vi "IMAQ FPGA CXP 8-Bit x 16.vi"(6 "Ready for Output":bool=TRUE, 7 "Reset":bool, 9 "Image Skip Count":u16, 10 "CXP Options":T1, 11 "CXP NI AXI4-S Bus":T3) -> (0 "Output Valid":bool, 2 "Acquisition Status":T2, 3 "Vision Pixel Bus Out":T4={"Pixel Data"=[0, 0, 0, 0, 0, 0, 0, 0, 0, 0, 0, 0, 0, 0, 0, 0], "DV"=[FALSE, FALSE, FALSE, FALSE, FALSE, FALSE, FALSE, FALSE, FALSE, FALSE, FALSE, FALSE, FALSE, FALSE, FALSE, FALSE], "EOL"=FALSE, "EOI"=FALSE, "Data Type"=enum."U8 x 16"}, 4 "Ready For Input":bool)   [LabVIEW 2020]
doc: "Acquires images from a CoaXPress camera. The VI converts the pixels from NI_AXI4-S format to Vision Pixel Bus containing 16 adjacent pixels. The <B>Vision Pixel Bus Out</B> can be connected to Vision FPGA algorithms for processing or transferred to the host. Ensure that this VI is called from a Single Cycle Timed Loop. Use multiple instances of this VI along with <B>Device ID</B> and <B>Stream ID</B> inputs to output a Vision Pixel Bus for multiple cameras."
uses:
  <vilib>/visionFPGA/Controls/IMAQ FPGA Pixel Bus u8x16.ctl
  <vilib>/visionFPGA/Basics/CoaXPress Acquisition/Controls/IMAQ FPGA CXP NI AXI4-S Bus.ctl
  <vilib>/visionFPGA/Basics/CoaXPress Acquisition/Controls/IMAQ FPGA CXP FPGA Options.ctl
  <vilib>/rvi/Emulation/niFpgaSctlEmulationGetInTimedLoop.vi
  <vilib>/Utility/error.llb/Clear Errors.vi
  <vilib>/rvi/DataTransferAndStorage/Container/Common/niFpgaContainerGetUniqueNameForEmu.vi
  <vilib>/rvi/DataTransferAndStorage/Container/Common/niFpgaContainerSetEmuInfo.vi
  <vilib>/rvi/eio/common/nirviEmuReportErrorAndStop.vi
  <vilib>/rvi/DataTransferAndStorage/Container/Common/niFpgaContainerExecOnDevCompGetState.vi
  <vilib>/rvi/Emulation/niFpgaEmulationIsFPGAContextNoSignature.vi
  <vilib>/rvi/errors/niFpgaSetErrorForExecOnDevCompSimple.vi
  <vilib>/rvi/FIFO/Fifo_Resource/nirvififoEmulationSetSize.vi
  <vilib>/rvi/FIFO/Fifo_Resource/nirviFifoEmulationQueueMgr.vi
  <instcachedir>/0/nirviFifoEmulationQueueMgr_E5CAEC123FF24DC58D834DCA3CDAA9B5.lvgen/nirviFifoEmulationQueueMgr_E5CAEC123FF24DC58D834DCA3CDAA9B5_008.vi
  <vilib>/rvi/FIFO/Fifo_Resource/nirvififoEmulationDetermineInputValidOut.vi
  <vilib>/rvi/FIFO/Fifo_Resource/nirvififoEmulationCreateLock.vi
  <vilib>/rvi/Emulation/niFpgaProcessEmulError.vi
  <vilib>/rvi/FIFO/Fifo_Resource/nirvififoEmulationObtainLock.vi
  <vilib>/rvi/FIFO/Fifo_Resource/nirvififoEmulationReleaseLock.vi
  <vilib>/rvi/occurrence/nirviWaitOnOccurrenceBase.vi
  <vilib>/rvi/errors/nirviReportUnexpectedCaseInternalError.vi
  <vilib>/rvi/errors/nirviReportUnexpectedCaseInternalError (U32).vi
  <vilib>/rvi/interface/RandomDataEmulation/niFpgaRandomDataHandleErrors.vi
  <vilib>/rvi/LocalResourceManager/LocalResourceManager.xnode
  <vilib>/rvi/DataTransferAndStorage/Container/XNode/niFpgaContainer.xnode
  <vilib>/rvi/FIFO/Fifo_Resource/niFpgaFifoEmulationRefIn.vi
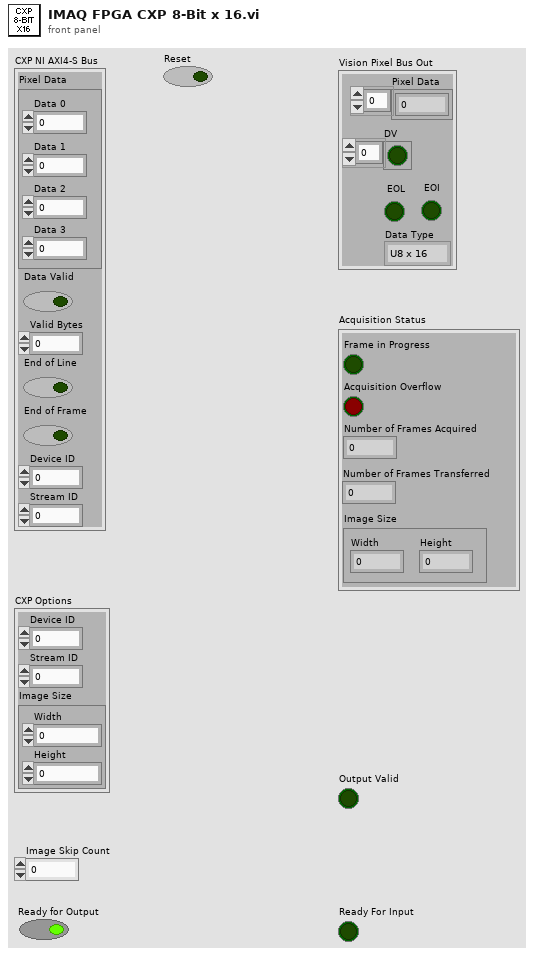
[diagram p1: front panel]
types:
  T1 = typedef "IMAQ FPGA CXP FPGA Options.ctl" = cluster{"Device ID":u8, "Stream ID":u8, "Image Size":cluster{"Width":u16, "Height":u16}}
  T2 = cluster{"Frame in Progress":bool, "Acquisition Overflow":bool, "Number of Frames Acquired":u64, "Number of Frames Transferred":u64, "Image Size":cluster{"Width":u16, "Height":u16}}
  T3 = typedef "IMAQ FPGA CXP NI AXI4-S Bus.ctl" = cluster{"Pixel Data":cluster{"Data 0":u64, "Data 1":u64, "Data 2":u64, "Data 3":u64}, "Data Valid":bool, "Valid Bytes":u8, "End of Line":bool, "End of Frame":bool, "Device ID":u8, "Stream ID":u8}
  T4 = typedef "IMAQ FPGA Pixel Bus u8x16.ctl" = cluster{"Pixel Data":u8[], "DV":bool[], "EOL":bool, "EOI":bool, "Data Type":enum16{"U8 x 16"}}
  T5 = cluster{"Pixel Data":cluster{"Data 0":u64, "Data 1":u64, "Data 2":u64, "Data 3":u64}, "Data Valid":bool, "Valid Bytes":u8, "End of Line":bool, "End of Frame":bool, "Device ID":u8, "Stream ID":u8}
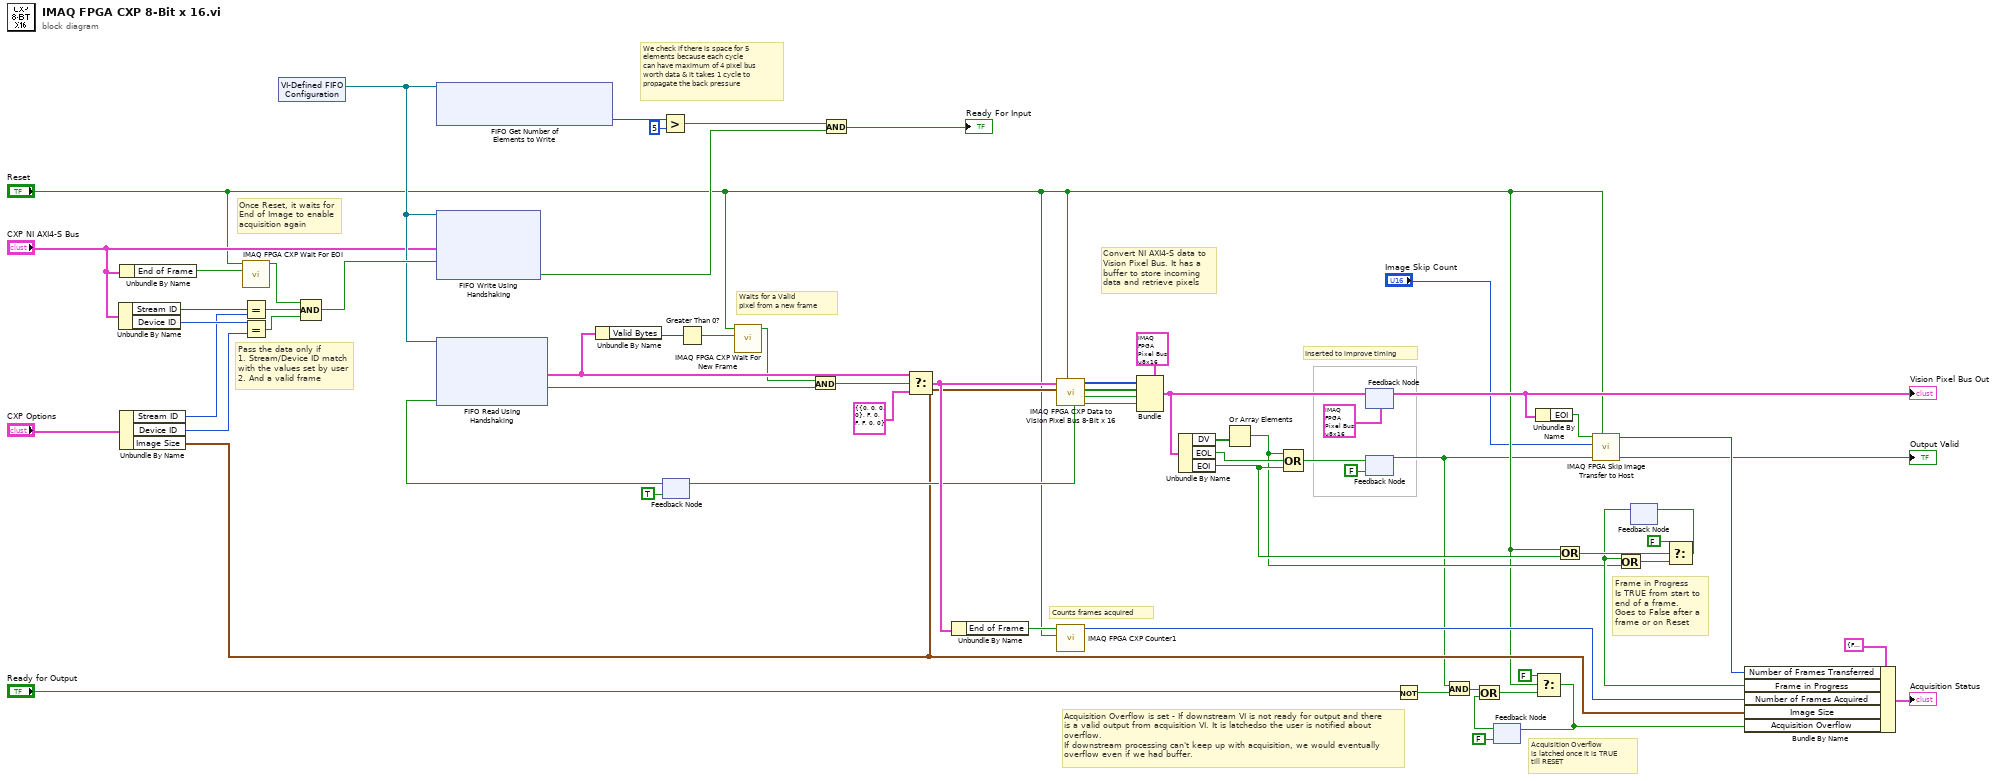
[diagram p0: block diagram]
diagram:
  # "We check if there is space for 5\nelements because each cycle\ncan have maximum of 4 pixel bus\nworth data & it takes 1 cycle to \npropagate the back pressure"
  # "Waits for a Valid\npixel from a new frame"
  # "Pass the data only if\n1. Stream/Device ID match\nwith the values set by user\n2. And a valid frame"
  # "Once Reset, it waits for\nEnd of Image to enable\nacquisition again"
  # "Frame in Progress\nIs TRUE from start to \nend of a frame. \nGoes to False after a\nframe or on Reset"
  # "Acquisition Overflow\nis latched once it is TRUE\ntill RESET"
  # "Convert NI AXI4-S data to\nVision Pixel Bus. It has a \nbuffer to store incoming\ndata and retrieve pixels"
  # "Counts frames acquired"
  # "Inserted to improve timing"
  # "Acquisition Overflow is set - If downstream VI is not ready for output and there \nis a valid output from acquisition VI. It is latchedso the user is notified about\noverflow. \nIf downstream processing can't keep up with acquisition, we would eventually \noverflow even if we had buffer."
  n1 = Unbundle By Name("CXP NI AXI4-S Bus") -> ("Stream ID"=w44:u8, "Device ID"=w43:u8)
  n2 = Unbundle By Name("CXP Options") -> ("Stream ID"=w12:u8, "Device ID"=w11:u8, "Image Size"=w10:cluster{"Width":u16, "Height":u16})
  n3 = Unbundle By Name("CXP NI AXI4-S Bus") -> ("End of Frame"=w23:bool)
  n4 = call <vilib>:"IMAQ FPGA CXP Wait For EOI.vi"("EOI"=w23, "Reset"="Reset") -> ("Enable"=w24:bool)  [unwired: 9 in]
  n5 = Equal?(x=w44, y=w12) -> (x = y?=w53:bool)
  n6 = Equal?(x=w43, y=w11) -> (x = y?=w52:bool)
  n7 = xnode "VI-Defined FIFO Configuration"() -> ("FIFO Out"=w36:refnum<k21>)
  n8 = Compound Arithmetic op=AND(w24, w53, w52) -> (w39:bool)
  n9 = xnode "FIFO Get Number of Elements to Write"("FIFO In"=w36) -> ("Number of Elements to Write"=w37:u32)  [unwired: 1 out]
  n10 = xnode "FIFO Write Using Handshaking"("Element"="CXP NI AXI4-S Bus", "Input Valid"=w39, "FIFO In"=w36) -> ("Ready for Input"=w21:bool)  [unwired: 1 out]
  n11 = Greater?(x=w37, y=u32 5) -> (0:w22:bool)
  n12 = feedback #1(TRUE ("Ready for Input")) -> (w34:bool)
  n13 = xnode "FIFO Read Using Handshaking"("Ready for Output"=w34, "FIFO In"=w36) -> ("Element"=w19:T5, "Output Valid"=w15:bool)  [unwired: 1 out]
  n14 = Unbundle By Name(w19) -> ("Valid Bytes"=w18:u8)
  n15 = Greater Than 0?(x=w18) -> (x > 0?=w17:bool)
  n16 = call <vilib>:"IMAQ FPGA CXP Wait For New Frame.vi"("DV"=w17, "Reset"="Reset") -> ("Enable"=w16:bool)  [unwired: 9 in]
  n17 = And(x=w16, y=w15) -> (x .and. y?=w14:bool)
  n18 = And(x=w22, y=w21) -> (x .and. y?=→"Ready For Input":bool)
  n19 = Select(t=w19, s=w14, f=T3 {"Pixel Data"={"Data 0"=0, "Data 1"=0, "Data 2"=0, "Data 3"=0}, "Data Valid"=FALSE, "Valid Bytes"=0, "End of Line"=FALSE, "End of Frame"=FALSE, "Device ID"=0, "Stream ID"=0} ("CXP NI AXI4-S Bus")) -> (s? t:f=w47:T3)
  n20 = Unbundle By Name(w47) -> ("End of Frame"=w49:bool)
  n21 = call <vilib>:"IMAQ FPGA CXP Data to Vision Pixel Bus 8-Bit x 16.vi"("Reset"="Reset", "Image Size"=w10, "CXP Data"=w47) -> ("EOI"=w61:bool, "EOL"=w62:bool, "DV"=w63:bool[], "Pixel Data"=w64:u8[], "Ready for Input"=w35:bool)  [unwired: 4 in]
  n22 = feedback-in #1(w35) -> ()
  n23 = call <vilib>:"IMAQ FPGA CXP Counter1.vi"("Reset"="Reset", "Increment"=w49) -> ("Count 1"=w48:u64)  [unwired: 9 in]
  n24 = Bundle(cluster=T4 {"Pixel Data"=[0, 0, 0, 0, 0, 0, 0, 0, 0, 0, 0, 0, 0, 0, 0, 0], "DV"=[FALSE, FALSE, FALSE, FALSE, FALSE, FALSE, FALSE, FALSE, FALSE, FALSE, FALSE, FALSE, FALSE, FALSE, FALSE, FALSE], "EOL"=FALSE, "EOI"=FALSE, "Data Type"=enum."U8 x 16"} ("Vision Pixel Bus Out"), "Pixel Data"=w64, "DV"=w63, "EOL"=w62, "EOI"=w61) -> (w60:T4)  [unwired: 1 in]
  n25 = Unbundle By Name(w60) -> ("DV"=w65:bool[], "EOL"=w66:bool, "EOI"=w27:bool)
  n26 = Or Array Elements(Boolean array=w65) -> (logical OR=w26:bool)
  n27 = Compound Arithmetic op=OR(w26, w66, w27) -> (w59:bool)
  n28 = feedback #2(T4 {"Pixel Data"=[0, 0, 0, 0, 0, 0, 0, 0, 0, 0, 0, 0, 0, 0, 0, 0], "DV"=[FALSE, FALSE, FALSE, FALSE, FALSE, FALSE, FALSE, FALSE, FALSE, FALSE, FALSE, FALSE, FALSE, FALSE, FALSE, FALSE], "EOL"=FALSE, "EOI"=FALSE, "Data Type"=enum."U8 x 16"} ("Vision Pixel Bus Out")) -> (w7:T4)
  "Vision Pixel Bus Out" <- w7
  n29 = feedback-in #2(w60) -> ()
  n30 = feedback #3(FALSE) -> (w3:bool)
  n31 = feedback-in #3(w59) -> ()
  n32 = Not(x="Ready for Output") -> (.not. x?=w58:bool)
  n33 = And(x=w3, y=w58) -> (x .and. y?=w57:bool)
  n34 = feedback #4(FALSE ("Reset Overflow")) -> (w50:bool)
  n35 = Compound Arithmetic op=OR(w57, w50) -> (w42:bool)
  n36 = Select(t=FALSE, s="Reset", f=w42) -> (s? t:f=w41:bool)
  n37 = feedback-in #4(w41) -> ()
  n38 = Unbundle By Name(w7) -> ("EOI"=w6:bool)
  n39 = Or(x="Reset", y=w27) -> (x .or. y?=w32:bool)
  n40 = call <vilib>:"IMAQ FPGA Skip Image Transfer to Host.vi"("Reset"="Reset", "Output Valid In"=w3, "Image Skip Count"="Image Skip Count", "EOI In"=w6) -> ("Output Valid Out"=→"Output Valid":bool, "Number of Frames Transferred"=w4:u64)  [unwired: 6 in]
  n41 = feedback #5() -> (w28:bool)  [unwired: 1 in]
  n42 = Or(x=w28, y=w26) -> (x .or. y?=w30:bool)
  n43 = Select(t=FALSE ("x .or. y?"), s=w32, f=w30) -> (s? t:f=w29:bool)
  n44 = feedback-in #5(w29) -> ()
  n45 = Bundle By Name(cluster=T2 {"Frame in Progress"=FALSE, "Acquisition Overflow"=FALSE, "Number of Frames Acquired"=0, "Number of Frames Transferred"=0, "Image Size"={"Width"=0, "Height"=0}} ("Acquisition Status"), "Number of Frames Transferred"=w4, "Frame in Progress"=w28, "Number of Frames Acquired"=w48, "Image Size"=w10, "Acquisition Overflow"=w41) -> (→"Acquisition Status":T2)
